vi "Spartan HTTP Generate Reply.vi"(4 "error in (no error)":errorcluster, 6 "request info":T3={"process"=FALSE, "accessed document"="", "request type"=enum."CGI Movie", "reply"={"content"="", "header"="", "keep alive"=FALSE, "don't write"=FALSE}, "script alias"=FALSE}, 7 "HTTP Data":T4 {"object data"."time" format="%0.2f"}) -> (0 "error out":errorcluster)   [LabVIEW 2011]
uses:
  Spartan HTTP Session.ctl
  Addons/internet/http/http_obj.llb/HTTP Session Data.ctl
  Addons/internet/utils/keyedarr.llb/Keyed Array.ctl
  Addons/internet/http/http1.llb/HTTP Request Type.ctl
  Addons/internet/http/cgi.llb/CGI Reply.ctl
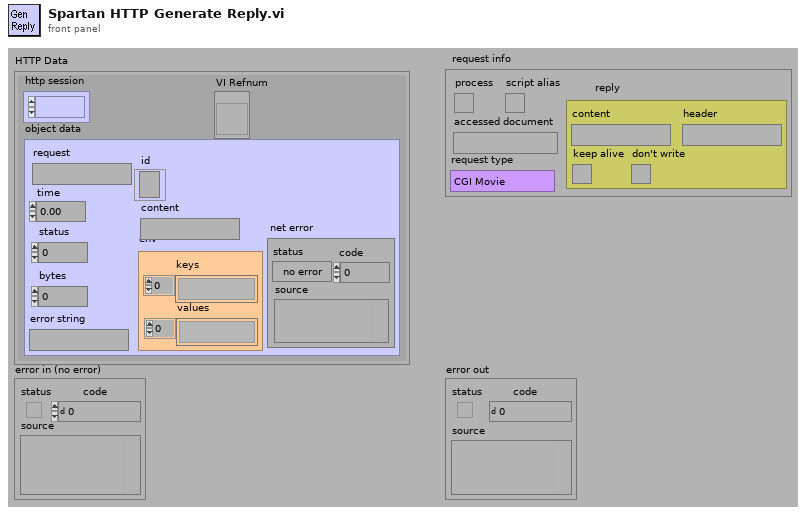
[diagram p1: front panel]
types:
  T1 = typedef "HTTP Request Type.ctl" = enum16{"Default", "Panel Picture", "Panel Movie", "CGI Movie"}
  T2 = typedef "CGI Reply.ctl" = cluster{"content":string, "header":string, "keep alive":bool, "don't write":bool}
  T3 = cluster{"process":bool, "accessed document":string, "request type":T1, "reply":T2, "script alias":bool}
  T4 = typedef "Spartan HTTP Session.ctl" = cluster{"http session":refnum<k1>, "object data":T5, "VI Refnum":refnum<vi>}
  T5 = typedef "HTTP Session Data.ctl" = cluster{"request":string, "time":dbl, "status":i32, "error string":string, "bytes":i32, "env":T6, "content":string, "id":refnum<k5>, "net error":errorcluster}
  T6 = typedef "Keyed Array.ctl" = cluster{"keys":string[], "values":string[]}
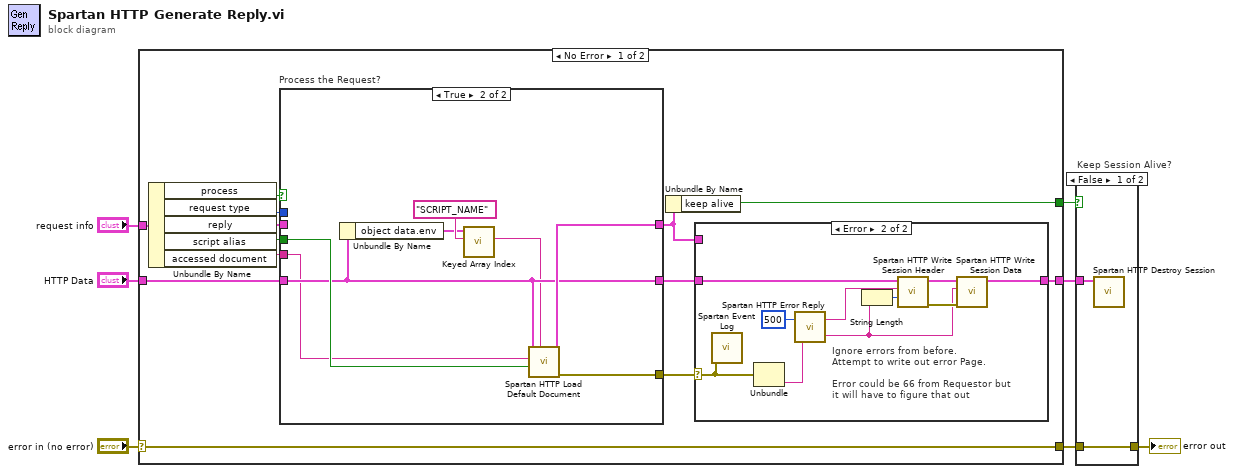
[diagram p0: block diagram]
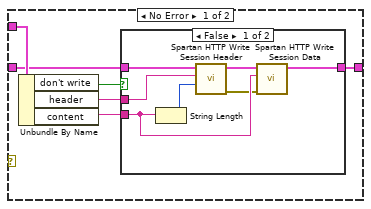
[diagram p4: hidden frame]
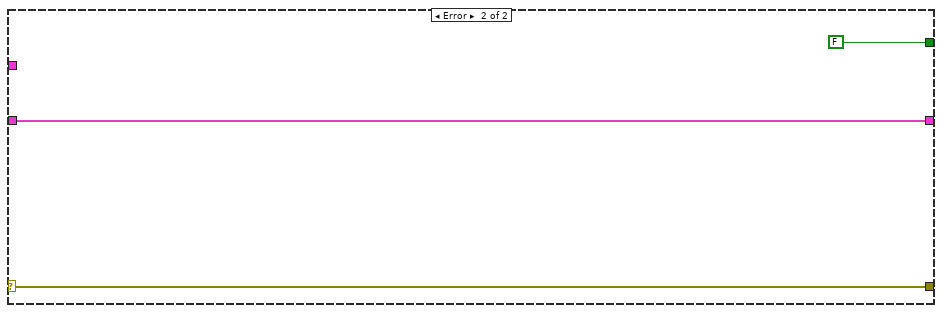
[diagram p6: hidden frame]
diagram:
  n1 = case shown="No Error" "error in (no error)" {
    selector: "error in (no error)" -> [w9 w55]
    tunnel: "HTTP Data" -> [w14 w56]
    tunnel: [w19 FALSE ("keep alive")] -> w6
    tunnel: [w10 w56] -> w7
    tunnel: [w9 w55] -> w2
    tunnel: "request info" -> [w12 _]
    frame No Error {
      n2 = Unbundle By Name(w12) -> ("process"=w18:bool, "request type"=w17:T1, "reply"=w16:T2, "script alias"=w11:bool, "accessed document"=w8:string)
      n3 = case "Process the Request?" shown="True" w18 {
        tunnel: [w21 w30] -> w20
        tunnel: w14 -> [w22 w27]
        tunnel: w16 -> [w21 _]
        tunnel: w17 -> [_ _]
        tunnel: w11 -> [_ w29]
        tunnel: [_ w28] -> w15
        tunnel: [w22 w27] -> w13
        tunnel: w8 -> [_ w26]
        frame False {
          # "This case might happen if the request\nwas determined already to be invalid, etc..."
        }
        frame True {
          n4 = Unbundle By Name(w27) -> ("object data.env"=w24:T6)
          n5 = call "Keyed Array Index.vi"("key"="SCRIPT_NAME" ("name"), "array in"=w24) -> ("value"=w23:string)  [unwired: 2 in, 3 out]
          n6 = call "Spartan HTTP Load Default Document.vi"("url path"=w23, "script alias"=w29, "absolut path"=w26, "HTTP Data"=w27) -> ("error out"=w28:errorcluster, "Reply"=w30:T2)  [unwired: 1 in, 5 out]
        }
      }
      n7 = Unbundle By Name(w20) -> ("keep alive"=w19:bool)
      n8 = case shown="Error" w15 {
        selector: w15 -> [_ w45]
        tunnel: w20 -> [w36 _]
        tunnel: [w32 w49] -> w10
        tunnel: w13 -> [w31 w54]
        frame No Error {
          n9 = Unbundle By Name(w36) -> ("don't write"=w35:bool, "header"=w34:string, "content"=w33:string)
          n10 = case shown="False" w35 {
            tunnel: w33 -> [w40 _]
            tunnel: w34 -> [w43 _]
            tunnel: [w37 w44] -> w32
            tunnel: w31 -> [w41 w44]
            frame False {
              n11 = String Length(string=w40) -> (length=w42:i32)
              n12 = call "Spartan HTTP Write Session Header.vi"("content length (-1)"=w42, "header"=w43, "http session"=w41) -> ("error out"=w39:errorcluster, "http session out"=w38:T4)  [unwired: 2 in, 5 out]
              n13 = call "Spartan HTTP Write Session Data.vi"("error in (no error)"=w39, "data"=w40, "http session"=w38) -> ("http session out"=w37:T4)  [unwired: 4 out]
            }
            frame True {
            }
          }
        }
        frame Error {
          # "Ignore errors from before.  \nAttempt to write out error Page.\n\nError could be 66 from Requestor but\nit will have to figure that out"
          n14 = call "Spartan Event Log.vi"("error in (no error)"=w45) -> ()  [unwired: 4 in, 4 out]
          n15 = Unbundle(w45) -> ("source"=w48:string)  [unwired: 2 out]
          n16 = call "Spartan HTTP Error Reply.vi"("message"=w48, "status code"=500) -> ("content"=w47:string, "header"=w53:string)
          n17 = String Length(string=w47) -> (length=w52:i32)
          n18 = call "Spartan HTTP Write Session Header.vi"("content length (-1)"=w52, "header"=w53, "http session"=w54) -> ("error out"=w50:errorcluster, "http session out"=w51:T4)  [unwired: 2 in, 5 out]
          n19 = call "Spartan HTTP Write Session Data.vi"("error in (no error)"=w50, "data"=w47, "http session"=w51) -> ("http session out"=w49:T4)  [unwired: 4 out]
        }
      }
    }
    frame Error {
    }
  }
  n20 = case "Keep Session Alive?" shown="False" w6 {
    tunnel: w7 -> [w58 _]
    tunnel: w2 -> [w59 w60]
    tunnel: [w59 w60] -> w1
    frame False {
      n21 = call "Spartan HTTP Destroy Session.vi"("object"=w58) -> ()  [unwired: 2 in, 9 out]
    }
    frame True {
    }
  }
  "error out" <- w1
